vi "Send Lock-in Command.vi"(6 "Context":T1, 7 "Message Priority (Normal)":T2=enum."Normal", 8 "error in (no error)":errorcluster, 10 "Lock-in":bool, 11 "Message Enqueuer":refnum<class "Message Enqueuer.lvclass">) -> (0 "error out":errorcluster, 3 "Message Enqueuer out":refnum<class "Message Enqueuer.lvclass">)   [LabVIEW 2021, in "Lock-in Command Msg.lvclass"]
doc: "This VI sends the message to an actor."
uses:
  Lock-in Command Msg.lvclass
  <vilib>/ActorFramework/Message Enqueuer/Message Enqueuer.lvclass
  <vilib>/ActorFramework/Message Enqueuer/Message Priority.ctl
  C:/Program Files/National Instruments/LabVIEW 2021/vi.lib/ActorFramework/Message/Message.lvclass
  Lock-in Command Msg.lvclass/Lock-in Command Msg.ctl
  <vilib>/ActorFramework/Message Enqueuer/Message Enqueuer.lvclass/Message Enqueuer.ctl
  <vilib>/ActorFramework/Message Priority Queue/Priority Enqueue.vi
  C:/GitHub/LabActor/Pulse Recorders/Lockin Digitizer Messages/Lock-in Command Msg/Lock-in Command Msg.lvclass
  Lockin Digitizer/L-D Command Context.ctl
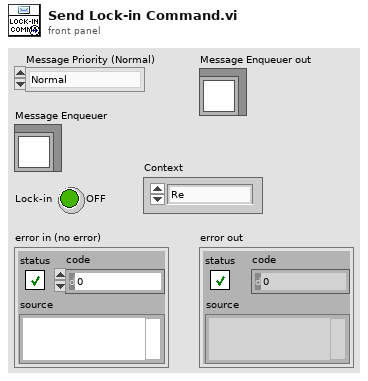
[diagram p1: front panel]
types:
  T1 = typedef "L-D Command Context.ctl" = enum16{"Re", "Switch", "Measure", "Arm"}
  T2 = typedef "Actor Framework.lvlib/Message Enqueuer.lvclass/Message Priority.ctl" = enum16{"Low", "Normal", "High"}
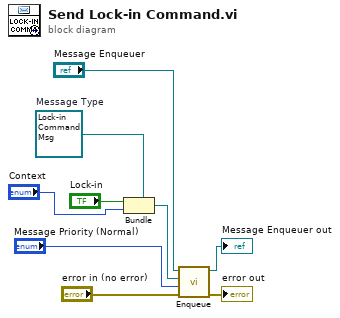
[diagram p0: block diagram]
diagram:
  w6 = refnum<class "Lock-in Command Msg.lvclass"> refnum  # Message Type
  n1 = Bundle(cluster=w6, "Lock-in", "Context") -> (w5:refnum<class "Lock-in Command Msg.lvclass">)
  n2 = call <vilib>:"Enqueue.vi"("error in (no error)"="error in (no error)", "Message Priority (Normal)"="Message Priority (Normal)", "Message"=w5, "Message Enqueuer in"="Message Enqueuer") -> ("error out"=→"error out":errorcluster, "Message Enqueuer out"=→"Message Enqueuer out":refnum<class "Message Enqueuer.lvclass">)  [unwired: 6 in]
